vi "Untitled 2.vi"() -> ()   [LabVIEW 2018]
panel:
  out "lo(x)":u8 format="%.0x"
  out "hi(x)":u8 format="%.0x"
  out "number":u8[](array[numeric]) format="%.0x"
  out "Array":string[](array[string])
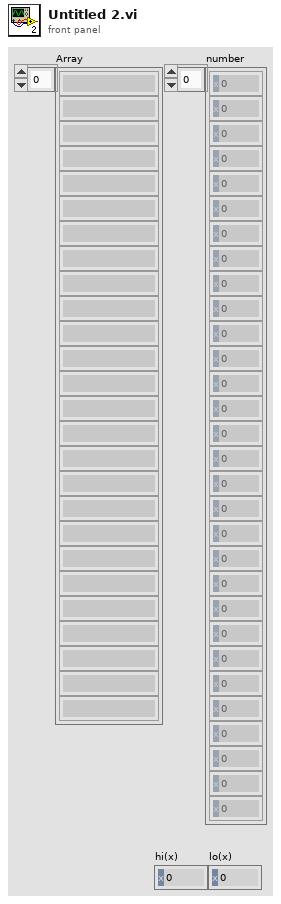
[diagram p1: front panel]
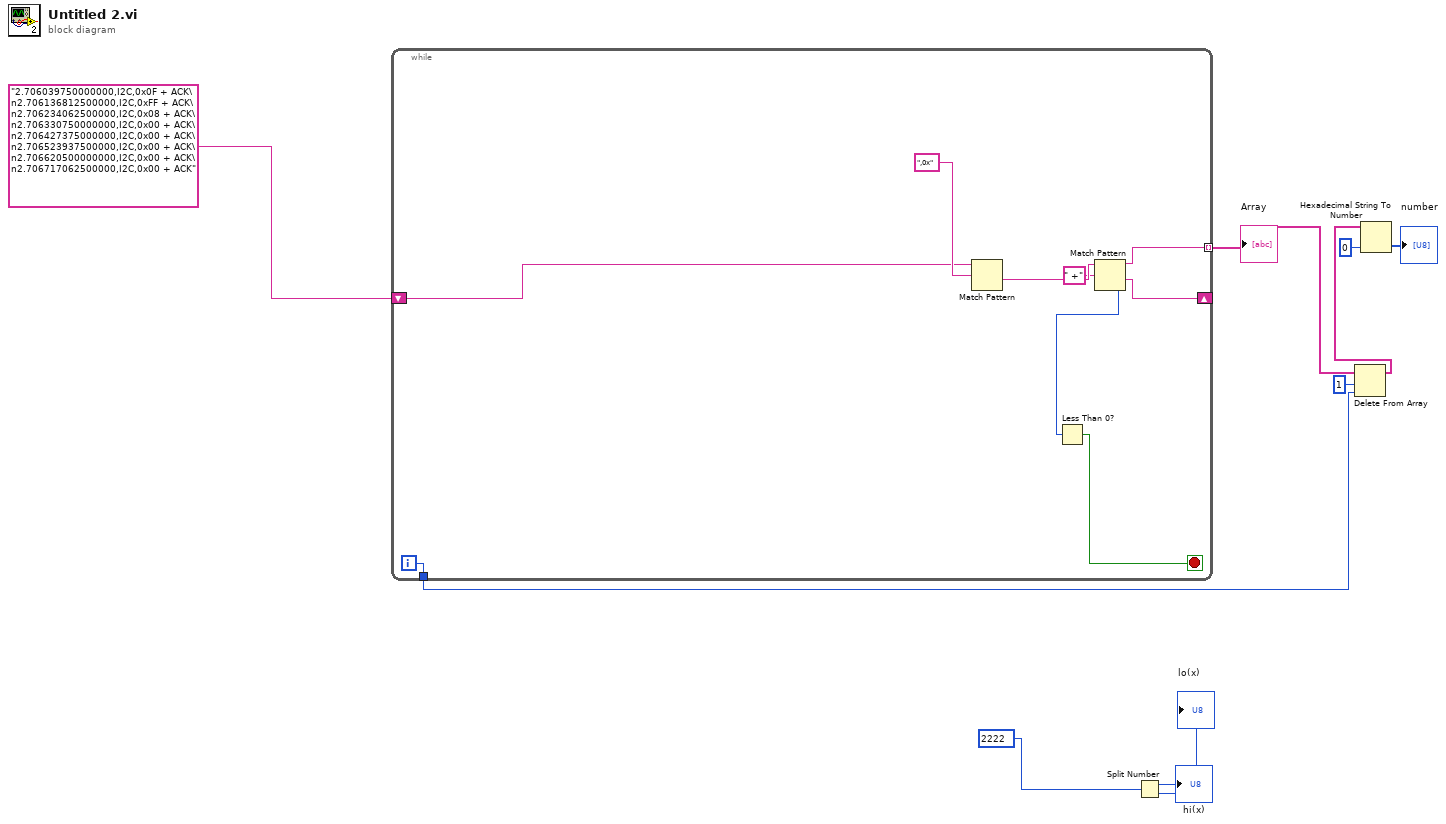
[diagram p0: block diagram]
diagram:
  n1 = while {
    shift-right: [w15] -> _
    shift-left: "2.706039750000000,I2C,0x0F + ACK\n2.706136812500000,I2C,0xFF + ACK\n2.706234062500000,I2C,0x08 + ACK\n2.706330750000000,I2C,0x00 + ACK\n2.706427375000000,I2C,0x00 + ACK\n2.706523937500000,I2C,0x00 + ACK\n2.706620500000000,I2C,0x00 + ACK\n2.706717062500000,I2C,0x00 + ACK" -> [w16]
    tunnel: [w14] -> w7 mode=indexing
    tunnel: [w11] -> w5
    i -> [w11]
    stop <- w12 stop-if-true
    n2 = Match Pattern(string=w16, regular expression=",0x" ("search string")) -> (after substring=w18:string)  [unwired: 1 in, 3 out]
    n3 = Match Pattern(string=w18, regular expression=" +") -> (before substring=w14:string, after substring=w15:string, offset past match=w13:i32)  [unwired: 1 in, 1 out]
    n4 = Less Than 0?(x=w13) -> (x < 0?=w12:bool)
  }
  "Array" <- w7
  n5 = Split Number(x=u16 2222) -> (hi(x)=→"hi(x)":u8, lo(x)=→"lo(x)":u8)
  n6 = Delete From Array(array=w7, length=1, index=w5) -> (array with subset deleted=w4:string[])  [unwired: 1 out]
  n7 = Hexadecimal String To Number(string=w4, default (0uL)=u32 0 ("default (0 U32)")) -> (number=→"number":u32[])  [unwired: 1 in, 1 out]
